vi "AvaSpec Main.vi"() -> ()   [LabVIEW 2013]
doc: "This Continuous Measurement sample project is based on the Queued Message Handler template.\n\nThe Event Handling Loop generates messages based on user interface actions.\n\nThe Message Handling Loop processes messages generated by the Event Handling Loop, or by other messages. There are also Acquisition and Logging message handling loop subVIs, and a chart updating loop."
uses:
  Acquisition/Color Parameters.ctl
  Settings/Settings.ctl
  Acquisition/Hardware Configuration.ctl
  Logging/Logging Configuration.ctl
  controls/AvaSpec UI Data.ctl
  controls/AvaSpec UI State.ctl
  support/Message Queue/Enqueue Message (Single).vi
  support/Message Queue/Enqueue Message (Array).vi
  <vilib>/Utility/error.llb/Error Cluster From Error Code.vi
  <vilib>/ErrorRing/Error Ring.xnode
  Acquisition/AvaSpec Acquisition.lvlib
  Logging/AvaSpec Logging.lvlib
  Settings/AvaSpec Settings.lvlib
  support/User Event - Stop/AvaSpec User Event - Stop.lvlib
  support/Message Queue/AvaSpec Message Queue.lvlib
panel:
  out "Color Parameters":T1
  in  "Settings":bool
  in  "Start":bool
  in  "Stop":bool
  out "Status":string
  in  "Exit":bool
  # "Continuous Measurement Data Logger"
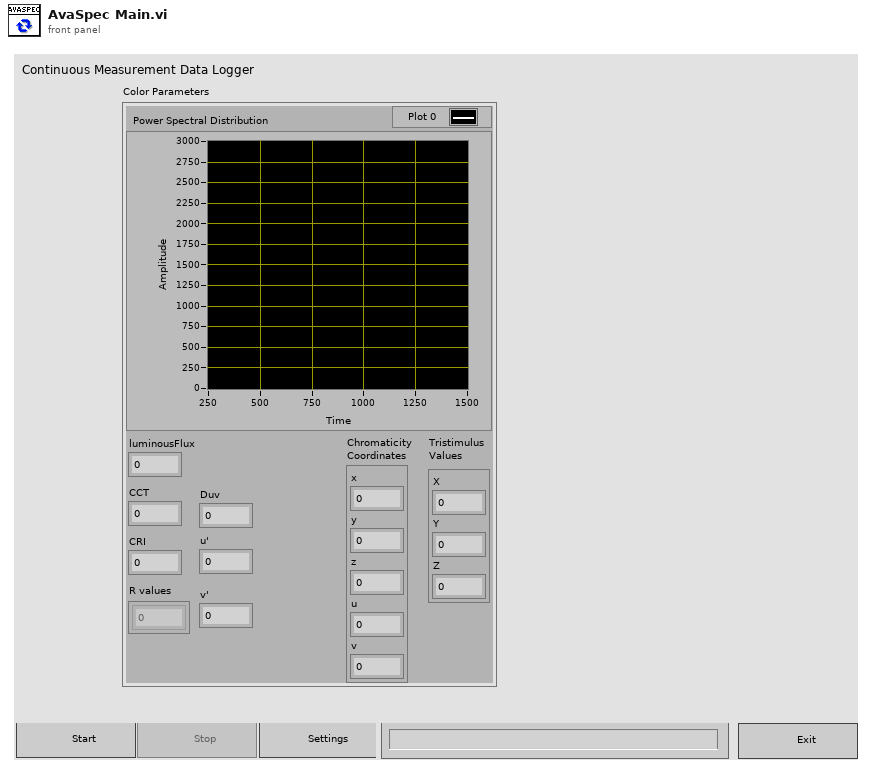
[diagram p1: front panel]
types:
  T1 = typedef "Color Parameters.ctl" = cluster{"Power Spectral Distribution":cluster{"X":dbl, "Y":dbl}[], "luminousFlux":dbl, "CCT":dbl, "CRI":dbl, "R values":dbl[], "Duv":dbl, "u'":dbl, "v'":dbl, "Chromaticity \nCoordinates":cluster{"x":dbl, "y":dbl, "z":dbl, "u":dbl, "v":dbl}, "Tristimulus \nValues":cluster{"X":dbl, "Y":dbl, "Z":dbl}}
  T2 = typedef "AvaSpec UI State.ctl" = enum16{"Idle", "Acquiring and Logging", "Waiting for Exit", "Waiting for Exit (Acq Stopped)", "Waiting for Exit (Log Stopped)", "Waiting for Stop", "Waiting for Stop (Acq Stopped)", "Waiting for Stop (Log Stopped)"}
  T3 = typedef "AvaSpec UI Data.ctl" = cluster{"Start Ref":refnum<vi>, "Stop Ref":refnum<vi>, "Settings Ref":refnum<vi>, "Exit Ref":refnum<vi>, "Status Ref":refnum<vi>, "Color Parameters":refnum<vi>}
  T4 = typedef "AvaSpec Settings.lvlib/Settings.ctl" = cluster{"Hardware Configuration":T5, "Logging Configuration":T6}
  T5 = typedef "AvaSpec Acquisition.lvlib/Hardware Configuration.ctl" = cluster{"Communication Settings":cluster{"Serial1":string, "Handle1":i32, "a_pDeviceId1":u8[], "a_pNumPixels":u16, "Port":i32, "a_hWnd":i32}, "a_pMeasConfig1":cluster{"StartPixel":u16, "StopPixel":u16, "IntTime":sgl, "IntDelay":u32, "NrOfAVG":u32, "DarkEnable":u8, "ForgetPercentage":u8, "SmoothPix":u16, "SmoothModel":u8, "SatDetection":u8, "TriggerMode":u8, "TriggerSource":u8, "TriggerSourceType":u8, "FlashesPerScan":u16, "LaserDelay":u32, "LaserWidth":u32, "LaserWavelenght":sgl, "RamSpectra":u16}}
  T6 = typedef "AvaSpec Logging.lvlib/Logging Configuration.ctl" = cluster{"Log File Base Path":path, "TDMS File Reference":refnum<k34>, "Calibration File Path":path, "Aux Correction File Path":path}
  T7 = typedef "AvaSpec Message Queue.lvlib/All Message Queues.ctl" = cluster{"UI":refnum<queue>, "Acquisition":refnum<queue>, "Logging":refnum<queue>}
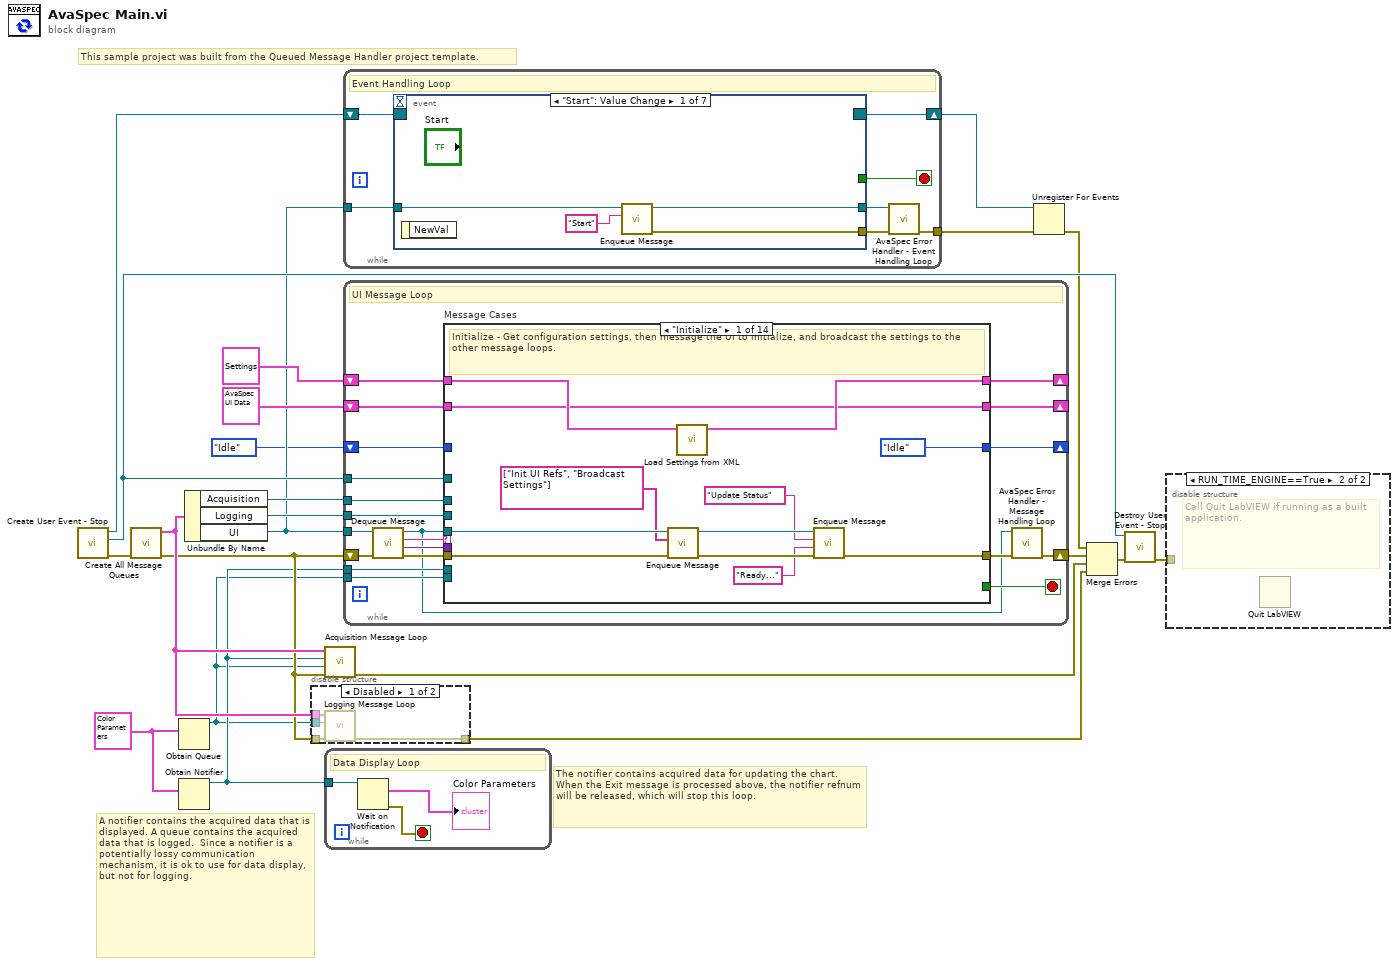
[diagram p0: block diagram]
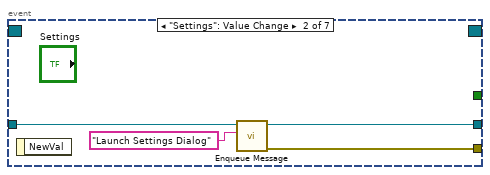
[diagram p4: hidden frame]
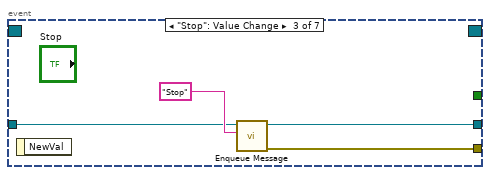
[diagram p5: hidden frame]
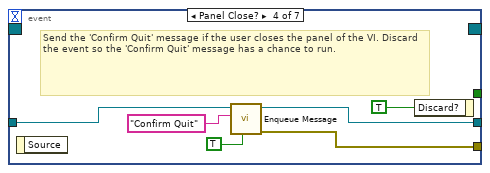
[diagram p6: hidden frame]
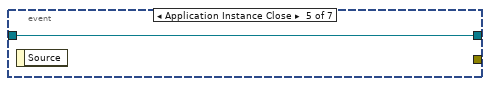
[diagram p7: hidden frame]
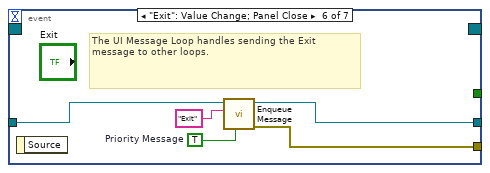
[diagram p8: hidden frame]
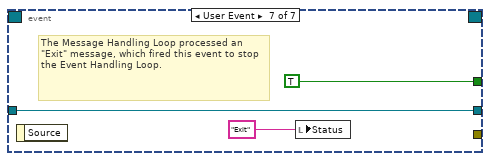
[diagram p9: hidden frame]
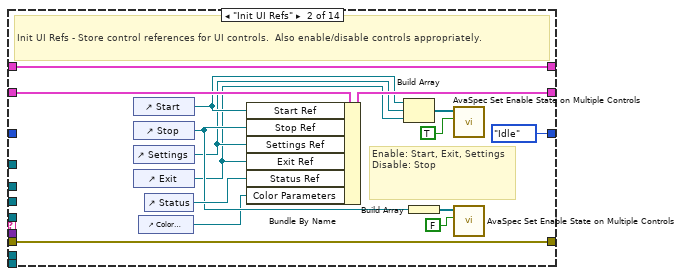
[diagram p10: hidden frame]
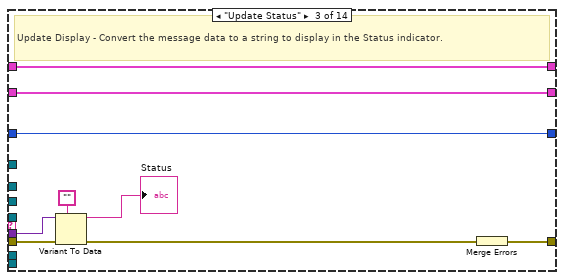
[diagram p11: hidden frame]
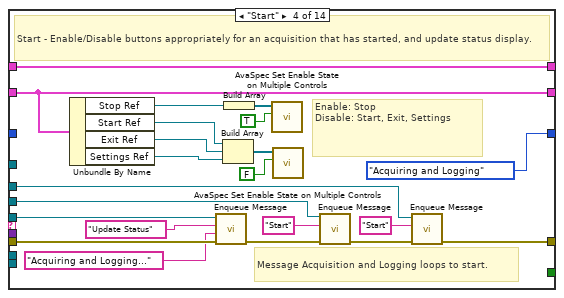
[diagram p12: hidden frame]
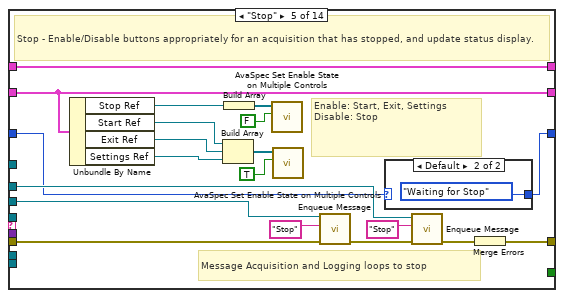
[diagram p13: hidden frame]
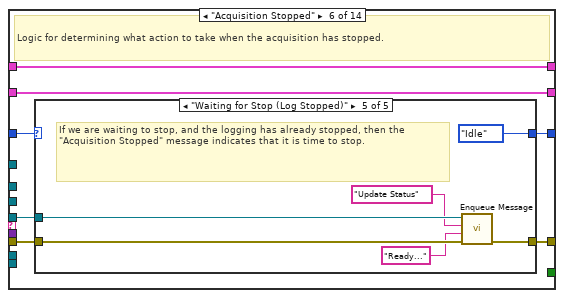
[diagram p15: hidden frame]
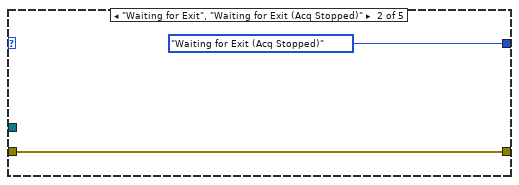
[diagram p17: hidden frame]
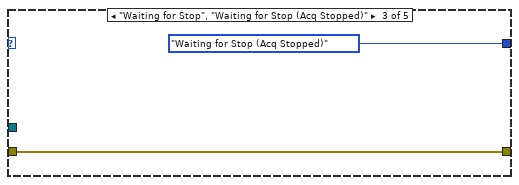
[diagram p18: hidden frame]
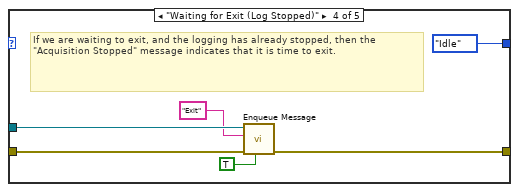
[diagram p19: hidden frame]
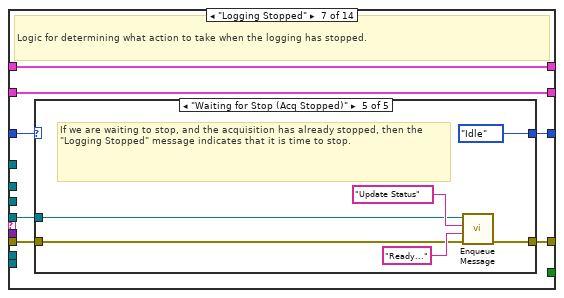
[diagram p20: hidden frame]
diagram:
  w1 = T1 {"Power Spectral Distribution"=[], "luminousFlux"=0.0, "CCT"=0.0, "CRI"=0.0, "R values"=[], "Duv"=0.0, "u'"=0.0, "v'"=0.0, "Chromaticity \nCoordinates"={"x"=0.0, "y"=0.0, "z"=0.0, "u"=0.0, "v"=0.0}, "Tristimulus \nValues"={"X"=0.0, "Y"=0.0, "Z"=0.0}} ("Color Parameters")
  # "This sample project was built from the Queued Message Handler project template."
  # "A notifier contains the acquired data that is displayed. A queue contains the acquired data that is logged.  Since a notifier is a potentially lossy communication mechanism, it is ok to use for data display, but not for logging."
  # "The notifier contains acquired data for updating the chart. When the Exit message is processed above, the notifier refnum will be released, which will stop this loop."
  n1 = call "Create User Event - Stop.vi"() -> ("error out"=w17:errorcluster, "User Event - Stop"=w19:refnum<user-event>, "Stop Event Registration Refnum"=w20:refnum<event-registration>)  [unwired: 9 in]
  n2 = call "Create All Message Queues.vi"("error in (no error)"=w17) -> ("error out"=w14:errorcluster, "Message Queues out"=w16:T7)  [unwired: 9 in]
  n3 = Obtain Queue(element data type=w1) -> (queue out=w2:refnum<queue>)  [unwired: 4 in, 2 out]
  n4 = Obtain Notifier(notification data type=w1) -> (notifier out=w3:refnum<notifier>)  [unwired: 3 in, 2 out]
  n5 = Unbundle By Name(w16) -> ("Acquisition"=w9:refnum<queue>, "Logging"=w8:refnum<queue>, "UI"=w7:refnum<queue>)
  n6 = disable-structure shown="Disabled" {
    disable-tunnel: w16 -> [w26 _]
    disable-tunnel: [w25 _] -> w15
    disable-tunnel: w14 -> [w24 _]
    disable-tunnel: w2 -> [w23 _]
    frame Disabled {
      n7 = call "Logging Message Loop.vi"("error in (no error)"=w24, "Data Queue"=w23, "Message Queues"=w26) -> ("error out"=w25:errorcluster)  [unwired: 8 in]
    }
    frame Enabled {
    }
  }
  n8 = call "Acquisition Message Loop.vi"("error in (no error)"=w14, "Data Queue"=w2, "Data Notifier"=w3, "Message Queues"=w16) -> ("error out"=w18:errorcluster)  [unwired: 7 in]
  n9 = while "Data Display Loop" {
    tunnel: w3 -> [w29]
    stop <- w28 stop-if-true
    # "Data Display Loop"
    n10 = Wait on Notification(notifier=w29) -> (notification=→"Color Parameters":T1, error out=w28:errorcluster)  [unwired: 3 in, 2 out]
  }
  n11 = while {
    tunnel: w7 -> [w35]
    tunnel: [w32] -> w21
    shift-right: [w34] -> w11
    shift-left: w20 -> [w36]
    stop <- w33 stop-if-true
    # "Event Handling Loop"
    n12 = event shown="[0] \"Start\": Value Change" {
      selector: w36 -> [_ _ _ _ _ _ _]
      dyn-events: [_ _ _ _ _ _ _] -> w34
      timeout: _ -> [_ _ _ _ _ _ _]
      tunnel: [_ _ _ _ _ _ TRUE ("Discard?")] -> w33
      tunnel: w35 -> [w40 w42 w47 w52 w55 w57 w61]
      tunnel: [w38 w44 w46 w50 _ w60 _] -> w31
      tunnel: [w37 w41 w45 w51 w55 w56 w61] -> w30
      event "Start": Value Change {
        n13 = event-data() -> ()  [unwired: 1 in, 1 out]
        n14 = call-poly "Enqueue Message.vi"("Message"="Start", "Message Queue"=w40) -> ("error out"=w38:errorcluster, "dup Message Queue"=w37:refnum<queue>)  [unwired: 8 in]
      }
      event "Settings": Value Change {
        n15 = event-data() -> ()  [unwired: 1 in, 1 out]
        n16 = call-poly "Enqueue Message.vi"("Message"="Launch Settings Dialog", "Message Queue"=w42) -> ("error out"=w44:errorcluster, "dup Message Queue"=w41:refnum<queue>)  [unwired: 8 in]
      }
      event "Stop": Value Change {
        n17 = event-data() -> ()  [unwired: 1 in, 1 out]
        n18 = call-poly "Enqueue Message.vi"("Message"="Stop", "Message Queue"=w47) -> ("error out"=w46:errorcluster, "dup Message Queue"=w45:refnum<queue>)  [unwired: 8 in]
      }
      event Panel Close? {
        # "Send the 'Confirm Quit' message if the user closes the panel of the VI. Discard the event so the 'Confirm Quit' message has a chance to run."
        n19 = event-data() -> ()  [unwired: 1 in, 1 out]
        n20 = call-poly "Enqueue Message.vi"("Priority Message? (F)"=TRUE, "Message"="Confirm Quit", "Message Queue"=w52) -> ("error out"=w50:errorcluster, "dup Message Queue"=w51:refnum<queue>)  [unwired: 7 in]
        n21 = event-data("Discard?"=TRUE) -> ()  [unwired: 1 in, 1 out]
      }
      event Application Instance Close {
        n22 = event-data() -> ()  [unwired: 1 in, 1 out]
      }
      event "Exit": Value Change; Panel Close {
        w58 = TRUE  # Priority Message
        # "The UI Message Loop handles sending the Exit message to other loops."
        n23 = event-data() -> ()  [unwired: 1 in, 1 out]
        n24 = call-poly "Enqueue Message.vi"("Priority Message? (F)"=w58, "Message"="Exit", "Message Queue"=w57) -> ("error out"=w60:errorcluster, "dup Message Queue"=w56:refnum<queue>)  [unwired: 7 in]
      }
      event User Event {
        # "The Message Handling Loop processed an \"Exit\" message, which fired this event to stop the Event Handling Loop."
        n25 = event-data() -> ()  [unwired: 1 in, 1 out]
        n26 = local write "Status"("Exit" ("Exit String")) -> ()
      }
    }
    n27 = call "AvaSpec Error Handler - Event Handling Loop.vi"("error in (no error)"=w31, "Message Queue"=w30) -> ("dup error in"=w32:errorcluster)  [unwired: 8 in, 1 out]
  }
  n28 = while {
    tunnel: w7 -> [w77]
    tunnel: w19 -> [w82]
    shift-right: [w68] -> w22
    shift-left: w14 -> [w81]
    shift-right: [w76] -> _
    shift-left: T4 {"Hardware Configuration"={"Communication Settings"={"Serial1"="", "Handle1"=0, "a_pDeviceId1"=[], "a_pNumPixels"=0, "Port"=0, "a_hWnd"=0}, "a_pMeasConfig1"={"StartPixel"=0, "StopPixel"=0, "IntTime"=0.0, "IntDelay"=0, "NrOfAVG"=0, "DarkEnable"=0, "ForgetPercentage"=0, "SmoothPix"=0, "SmoothModel"=0, "SatDetection"=0, "TriggerMode"=0, "TriggerSource"=0, "TriggerSourceType"=0, "FlashesPerScan"=0, "LaserDelay"=0, "LaserWidth"=0, "LaserWavelenght"=0.0, "RamSpectra"=0}}, "Logging Configuration"={"Log File Base Path"=path "", "TDMS File Reference"=refnum, "Calibration File Path"=path "", "Aux Correction File Path"=path ""}} ("Settings") -> [w75]
    shift-right: [w73] -> _
    shift-left: T3 {"Start Ref"=refnum, "Stop Ref"=refnum, "Settings Ref"=refnum, "Exit Ref"=refnum, "Status Ref"=refnum, "Color Parameters"=refnum} ("Measurement UI Controls") -> [w74]
    tunnel: w9 -> [w72]
    tunnel: w8 -> [w71]
    tunnel: w3 -> [w70]
    tunnel: w2 -> [w69]
    shift-right: [w64] -> _
    shift-left: AvaSpec_UI_State."Idle" ("UI State") -> [w65]
    stop <- w83 stop-if-true
    # "UI Message Loop"
    n29 = call "Dequeue Message.vi"("error in (no error)"=w81, "Message Queue"=w77) -> ("error out"=w80:errorcluster, "Message Data"=w78:variant, "Message"=w79:string, "dup Message Queue"=w66:refnum<queue>)  [unwired: 6 in]
    n30 = case "Message Cases" shown="\"Initialize\"" w79 {
      selector: w79 -> [_ _ _ _ _ _ _ _ _ _ _ _ _ w304]
      tunnel: w66 -> [w87 _ _ w141 _ w166 w191 _ w231 w245 w256 w287 _ _]
      tunnel: w80 -> [w86 w110 w118 w140 w160 w167 w192 w219 w233 w248 w255 w295 w302 _]
      tunnel: [w91 w110 w119 w123 w161 w164 w189 w225 w228 w244 w254 w296 w301 w303] -> w67
      tunnel: [_ _ _ _ _ _ _ _ _ _ _ TRUE _ _] -> w83
      tunnel: w78 -> [_ _ w117 _ _ _ _ _ _ w246 _ _ _ _]
      tunnel: w82 -> [_ _ _ _ _ _ _ _ _ _ _ w294 _ _]
      tunnel: [w94 w109 w113 w139 w159 w170 w195 w223 w230 w252 w259 w292 w300 w307] -> w76
      tunnel: w75 -> [w95 w109 w113 w139 w159 w170 w195 w223 w234 w252 w259 w292 w300 w307]
      tunnel: w74 -> [w88 w108 w112 w136 w158 w169 w194 w217 w227 w251 w258 w290 w299 w306]
      tunnel: [w88 w106 w112 w136 w158 w169 w194 w217 w227 w251 w258 w290 w299 w306] -> w73
      tunnel: w72 -> [_ _ _ w122 w145 _ _ w216 _ _ _ w289 _ _]
      tunnel: w71 -> [_ _ _ w125 w148 _ _ w215 _ _ _ w288 _ _]
      tunnel: w70 -> [_ _ _ _ _ _ _ _ _ _ _ w286 _ _]
      tunnel: w69 -> [_ _ _ _ _ _ _ _ _ _ _ w282 _ _]
      tunnel: w65 -> [_ _ w111 _ w142 w168 w193 w214 w226 w240 w257 _ w298 w305]
      tunnel: [AvaSpec_UI_State."Idle" ("UI State") AvaSpec_UI_State."Idle" ("UI State") w111 AvaSpec_UI_State."Acquiring and Logging" ("UI State") w143 w165 w190 w214 w226 w240 w253 AvaSpec_UI_State."Idle" ("UI State") w298 w305] -> w64
      frame "Initialize" {
        # "Initialize - Get configuration settings, then message the UI to initialize, and broadcast the settings to the other message loops."
        n31 = call-poly "Enqueue Message.vi"("error in (no error)"=w86, "Message Array"=string[] ["Init UI Refs", "Broadcast Settings"], "Message Queue"=w87) -> ("error out"=w93:errorcluster, "dup Message Queue"=w92:refnum<queue>)  [unwired: 7 in]
        n32 = call "Load Settings from XML.vi"("Settings in"=w95) -> ("Settings out"=w94:T4)  [unwired: 9 in, 1 out]
        n33 = call-poly "Enqueue Message.vi"("error in (no error)"=w93, "Message Data"="Ready..." ("Ready..."), "Message"="Update Status", "Message Queue"=w92) -> ("error out"=w91:errorcluster)  [unwired: 6 in, 1 out]
      }
      frame "Init UI Refs" {
        # "Enable: Start, Exit, Settings\nDisable: Stop"
        # "Init UI Refs - Store control references for UI controls.  Also enable/disable controls appropriately."
        n34 = control-ref of="Start"() -> (w100:refnum<vi>)
        n35 = control-ref of="Stop"() -> (w101:refnum<vi>)
        n36 = control-ref of="Settings"() -> (w99:refnum<vi>)
        n37 = control-ref of="Exit"() -> (w98:refnum<vi>)
        n38 = control-ref of="Color Parameters"() -> (w96:refnum<vi>)
        n39 = control-ref of="Status"() -> (w107:refnum<vi>)
        n40 = Bundle By Name(cluster=w108, "Start Ref"=w100, "Stop Ref"=w101, "Settings Ref"=w99, "Exit Ref"=w98, "Status Ref"=w107, "Color Parameters"=w96) -> (w106:T3)
        n41 = Build Array(w100, w99, w98) -> (w104:refnum<vi>[])
        n42 = Build Array(w101) -> (w103:refnum<vi>[])
        n43 = call "AvaSpec Set Enable State on Multiple Controls.vi"("Enable?"=TRUE, "Controls"=w104) -> ()  [unwired: 10 in]
        n44 = call "AvaSpec Set Enable State on Multiple Controls.vi"("Enable?"=FALSE, "Controls"=w103) -> ()  [unwired: 10 in]
      }
      frame "Update Status" {
        # "Update Display - Convert the message data to a string to display in the Status indicator."
        n45 = Variant To Data(error in=w118, type="", Variant=w117) -> (data=→"Status":string, error out=w115:errorcluster)
        n46 = Merge Errors(w115) -> (w119:errorcluster)
      }
      frame "Start" {
        # "Message Acquisition and Logging loops to start."
        # "Enable: Stop\nDisable: Start, Exit, Settings"
        # "Start - Enable/Disable buttons appropriately for an acquisition that has started, and update status display."
        n47 = Unbundle By Name(w136) -> ("Stop Ref"=w131:refnum<vi>, "Start Ref"=w130:refnum<vi>, "Exit Ref"=w129:refnum<vi>, "Settings Ref"=w128:refnum<vi>)
        n48 = call-poly "Enqueue Message.vi"("error in (no error)"=w140, "Message Data"="Acquiring and Logging..." ("Acquiring and Logging..."), "Message"="Update Status", "Message Queue"=w141) -> ("error out"=w127:errorcluster)  [unwired: 6 in, 1 out]
        n49 = Build Array(w130, w129, w128) -> (w134:refnum<vi>[])
        n50 = Build Array(w131) -> (w133:refnum<vi>[])
        n51 = call "AvaSpec Set Enable State on Multiple Controls.vi"("Enable?"=TRUE, "Controls"=w133) -> ()  [unwired: 10 in]
        n52 = call "AvaSpec Set Enable State on Multiple Controls.vi"("Enable?"=FALSE, "Controls"=w134) -> ()  [unwired: 10 in]
        n53 = call-poly "Enqueue Message.vi"("error in (no error)"=w127, "Message"="Start", "Message Queue"=w125) -> ("error out"=w124:errorcluster)  [unwired: 7 in, 1 out]
        n54 = call-poly "Enqueue Message.vi"("error in (no error)"=w124, "Message"="Start", "Message Queue"=w122) -> ("error out"=w123:errorcluster)  [unwired: 7 in, 1 out]
      }
      frame "Stop" {
        # "Message Acquisition and Logging loops to stop"
        # "Enable: Start, Exit, Settings\nDisable: Stop"
        # "Stop - Enable/Disable buttons appropriately for an acquisition that has stopped, and update status display."
        n55 = Unbundle By Name(w158) -> ("Stop Ref"=w153:refnum<vi>, "Start Ref"=w152:refnum<vi>, "Exit Ref"=w151:refnum<vi>, "Settings Ref"=w150:refnum<vi>)
        n56 = Build Array(w152, w151, w150) -> (w156:refnum<vi>[])
        n57 = Build Array(w153) -> (w155:refnum<vi>[])
        n58 = call "AvaSpec Set Enable State on Multiple Controls.vi"("Enable?"=FALSE, "Controls"=w155) -> ()  [unwired: 10 in]
        n59 = call "AvaSpec Set Enable State on Multiple Controls.vi"("Enable?"=TRUE, "Controls"=w156) -> ()  [unwired: 10 in]
        n60 = call-poly "Enqueue Message.vi"("error in (no error)"=w160, "Message"="Stop", "Message Queue"=w148) -> ("error out"=w147:errorcluster)  [unwired: 7 in, 1 out]
        n61 = case shown="Default" w142 {
          selector: w142 -> [w162 _]
          tunnel: [w162 AvaSpec_UI_State."Waiting for Stop" ("UI State")] -> w143
          frame "Waiting for Exit" {
          }
          frame Default {
          }
        }
        n62 = call-poly "Enqueue Message.vi"("error in (no error)"=w147, "Message"="Stop", "Message Queue"=w145) -> ("error out"=w146:errorcluster)  [unwired: 7 in, 1 out]
        n63 = Merge Errors(w146) -> (w161:errorcluster)
      }
      frame "Acquisition Stopped" {
        # "Logic for determining what action to take when the acquisition has stopped."
        n64 = case shown="\"Waiting for Stop (Log Stopped)\"" w168 {
          selector: w168 -> [w172 _ _ _ _]
          tunnel: w167 -> [w171 w174 w176 w182 w188]
          tunnel: w166 -> [_ _ _ w180 w185]
          tunnel: [w172 AvaSpec_UI_State."Waiting for Exit (Acq Stopped)" ("UI State") AvaSpec_UI_State."Waiting for Stop (Acq Stopped)" ("UI State") AvaSpec_UI_State."Idle" ("UI State") AvaSpec_UI_State."Idle" ("UI State")] -> w165
          tunnel: [w171 w174 w176 w181 w186] -> w164
          frame Default {
          }
          frame "Waiting for Exit", "Waiting for Exit (Acq Stopped)" {
          }
          frame "Waiting for Stop", "Waiting for Stop (Acq Stopped)" {
          }
          frame "Waiting for Exit (Log Stopped)" {
            # "If we are waiting to exit, and the logging has already stopped, then the \"Acquisition Stopped\" message indicates that it is time to exit."
            n65 = call-poly "Enqueue Message.vi"("Priority Message? (F)"=TRUE, "error in (no error)"=w182, "Message"="Exit", "Message Queue"=w180) -> ("error out"=w181:errorcluster)  [unwired: 6 in, 1 out]
          }
          frame "Waiting for Stop (Log Stopped)" {
            # "If we are waiting to stop, and the logging has already stopped, then the \"Acquisition Stopped\" message indicates that it is time to stop."
            n66 = call-poly "Enqueue Message.vi"("error in (no error)"=w188, "Message Data"="Ready..." ("Ready..."), "Message"="Update Status", "Message Queue"=w185) -> ("error out"=w186:errorcluster)  [unwired: 6 in, 1 out]
          }
        }
      }
      frame "Logging Stopped" {
        # "Logic for determining what action to take when the logging has stopped."
        n67 = case shown="\"Waiting for Stop (Acq Stopped)\"" w193 {
          selector: w193 -> [w197 _ _ _ _]
          tunnel: w192 -> [w196 w199 w201 w207 w210]
          tunnel: w191 -> [_ _ _ w205 w209]
          tunnel: [w197 AvaSpec_UI_State."Waiting for Exit (Log Stopped)" ("UI State") AvaSpec_UI_State."Waiting for Stop (Log Stopped)" ("UI State") AvaSpec_UI_State."Idle" ("UI State") AvaSpec_UI_State."Idle" ("UI State")] -> w190
          tunnel: [w196 w199 w201 w206 w208] -> w189
          frame Default {
          }
          frame "Waiting for Exit", "Waiting for Exit (Log Stopped)" {
          }
          frame "Waiting for Stop", "Waiting for Stop (Log Stopped)" {
          }
          frame "Waiting for Exit (Acq Stopped)" {
            # "If we are waiting to exit, and the acquisition has already stopped, then the \"Logging Stopped\" message indicates that it is time to exit."
            n68 = call-poly "Enqueue Message.vi"("Priority Message? (F)"=TRUE, "error in (no error)"=w207, "Message"="Exit", "Message Queue"=w205) -> ("error out"=w206:errorcluster)  [unwired: 6 in, 1 out]
          }
          frame "Waiting for Stop (Acq Stopped)" {
            # "If we are waiting to stop, and the acquisition has already stopped, then the \"Logging Stopped\" message indicates that it is time to stop."
            n69 = call-poly "Enqueue Message.vi"("error in (no error)"=w210, "Message Data"="Ready..." ("Ready..."), "Message"="Update Status", "Message Queue"=w209) -> ("error out"=w208:errorcluster)  [unwired: 6 in, 1 out]
          }
        }
      }
      frame "Broadcast settings" {
        w218 = "Update Settings" ("Message")
        # "Broadcast settings - Send the 'Update Settings' message to the Logging and Acquisition message loops."
        n70 = Unbundle By Name(w223) -> ("Hardware Configuration"=w222:T5, "Logging Configuration"=w221:T6)
        n71 = call-poly "Enqueue Message.vi"("Message Data"=w222, "Message"=w218, "Message Queue"=w216) -> ("error out"=w224:errorcluster)  [unwired: 7 in, 1 out]
        n72 = call-poly "Enqueue Message.vi"("error in (no error)"=w224, "Message Data"=w221, "Message"=w218, "Message Queue"=w215) -> ("error out"=w220:errorcluster)  [unwired: 6 in, 1 out]
        n73 = Merge Errors(w220, w219) -> (w225:errorcluster)
      }
      frame "Launch Settings Dialog" {
        # "Launch Settings Dialog - Launch the Settings Dialog when the user clicks the 'Settings' button."
        n74 = call "Settings Dialog.vi"("error in (no error)"=w233, "Settings in"=w234) -> ("error out"=w229:errorcluster, "Cancelled?"=w232:bool, "Settings out"=w230:T4)  [unwired: 6 in, 1 out]
        n75 = case shown="False" w232 {
          tunnel: w231 -> [w238 _]
          tunnel: w229 -> [w237 w239]
          tunnel: [w236 w239] -> w228
          frame False {
            n76 = call-poly "Enqueue Message.vi"("error in (no error)"=w237, "Message"="Broadcast Settings", "Message Queue"=w238) -> ("error out"=w236:errorcluster)  [unwired: 7 in, 1 out]
          }
          frame True {
          }
        }
      }
      frame "Error" {
        # "Error - Check the error message data and respond accordingly. This message is sent by the \"Error Handler\" VIs at the end of each loop in this application."
        n77 = Variant To Data(error in=w248, type=errorcluster {"status"=FALSE, "code"=0, "source"=""} ("error constant"), Variant=w246) -> (data=w250:errorcluster, error out=w247:errorcluster)
        n78 = call <vilib>:"Simple Error Handler.vi"("error in (no error)"=w250) -> ()  [unwired: 4 in, 5 out]
        n79 = call-poly "Enqueue Message.vi"("Priority Message? (F)"=TRUE, "Message"="Exit", "Message Queue"=w245) -> ("error out"=w243:errorcluster)  [unwired: 7 in, 1 out]
        n80 = Merge Errors(w243, w247) -> (w244:errorcluster)
      }
      frame "Confirm Quit" {
        # "Confirm Quit - Message that can confirm whether or not the user wants to exit the application."
        n81 = case shown="\"Acquiring and Logging\"" w257 {
          tunnel: w256 -> [w265 w269]
          tunnel: w255 -> [w264 w268]
          tunnel: [w263 w267] -> w254
          tunnel: [AvaSpec_UI_State."Idle" ("UI State") w266] -> w253
          frame Default {
            # "If 'Confirm Quit' comes in while the system is idle, there is no need for a confirmation message."
            n82 = call-poly "Enqueue Message.vi"("Priority Message? (F)"=TRUE, "error in (no error)"=w264, "Message"="Exit", "Message Queue"=w265) -> ("error out"=w263:errorcluster)  [unwired: 6 in, 1 out]
          }
          frame "Acquiring and Logging" {
            n83 = Two Button Dialog(message="Are you sure you want to quit while the acquisition is running?" ("Confirm Quit Message"), 1:"No" ("No"), 2:"Yes" ("Yes")) -> (T button?=w270:bool)
            n84 = case shown="True" w270 {
              tunnel: w269 -> [_ w279]
              tunnel: w268 -> [w275 w280]
              tunnel: [w275 w278] -> w267
              tunnel: [AvaSpec_UI_State."Acquiring and Logging" ("UI State") AvaSpec_UI_State."Waiting for Exit" ("UI State")] -> w266
              frame False {
                # "User did not want to quit."
              }
              frame True {
                n85 = call-poly "Enqueue Message.vi"("error in (no error)"=w280, "Message"="Stop", "Message Queue"=w279) -> ("error out"=w278:errorcluster)  [unwired: 7 in, 1 out]
              }
            }
          }
        }
      }
      frame "Exit" {
        w291 = "Exit" ("Message")
        # "Don't check the error outs. The acquisition and logging queues may have already been released."
        # "Close references owned by the Main VI."
        # "Stop the VI"
        # "Exit - Fire the User Event to stop the Event Handling Loop.  Also send Exit messages to the Acquisition and Logging loops."
        n86 = Release Queue(queue=w287, error in (no error)=w295) -> (error out=w285:errorcluster)  [unwired: 1 in, 2 out]
        n87 = call "Fire User Event - Stop.vi"("User Event - Stop"=w294) -> ("error out"=w293:errorcluster)  [unwired: 10 in]
        n88 = Release Notifier(notifier=w286, error in (no error)=w285) -> (error out=w284:errorcluster)  [unwired: 1 in, 2 out]
        n89 = Release Queue(queue=w282, error in (no error)=w284) -> (error out=w283:errorcluster)  [unwired: 1 in, 2 out]
        n90 = call-poly "Enqueue Message.vi"("Message"=w291, "Message Queue"=w289) -> ()  [unwired: 8 in, 2 out]
        n91 = call-poly "Enqueue Message.vi"("Message"=w291, "Message Queue"=w288) -> ()  [unwired: 8 in, 2 out]
        n92 = Merge Errors(w293, w283) -> (w296:errorcluster)
      }
      frame "---Copy This Frame---" {
        # "Duplicate this frame when creating new messages.  Change this comment in the duplicated frame to describe this message."
        n93 = Merge Errors(w302) -> (w301:errorcluster)
      }
      frame Default {
        # "'Default' case only runs if there is a message that isn't defined in any of the other cases.  Output a programming error."
        n94 = xnode "Error Ring"("parameter 0"=w304) -> ("error out"=w303:errorcluster)
      }
    }
    n95 = call "AvaSpec Error Handler - Message Handling Loop.vi"("error in (no error)"=w67, "Message Queue"=w66) -> ("dup error in"=w68:errorcluster)  [unwired: 8 in, 1 out]
  }
  n96 = Unregister For Events(event registration refnum=w11, error in=w21) -> (error out=w12:errorcluster)
  n97 = Merge Errors(w12, w22, w18, w15) -> (w4:errorcluster)
  n98 = call "Destroy User Event - Stop.vi"("error in (no error)"=w4, "User Event - Stop"=w19) -> ("error out"=w6:errorcluster)  [unwired: 9 in]
  n99 = disable-structure shown="RUN_TIME_ENGINE==True" {
    disable-tunnel: w6 -> [_ _]
    frame condition #0 (active) {
    }
    frame condition #1 {
      # "Call Quit LabVIEW if running as a built application."
      n100 = Quit LabVIEW() -> ()  [unwired: 1 in]
    }
  }
